vi "check limit channels.vi"(7 "RT Queues in":T8, 8 "Active channels":dbl[][](array[numeric]), 10 "Data":T1={"Parameters"={"FPGA Ref"=refnum, "data stream"={"data writer name"="error writer", "NS write buffer size"=16, "NS Buffer length"=0}, "FIFO Depth"=0, "Channel controls"={"FIFO channel count"=0, "active indices"=[], "active channels"=0, "channelScaling"=[], "scanivalveCount"=0, "channels"=[]}, "safetyChannels"={"oilP"=0, "airP"=0, "water"=0, "channelLimits"=[]}, "speedChannel"=0, "maxSpeedLimit"=0.0, "Torque"={"fixedOffset"=0.0, "filter"=FALSE, "fallingEdge"=FALSE, "swapEncoders"=FALSE}}, "Variables"={"Intermediary buffer"=[], "buffer position"=0, "write loop counter"=0, "NS write trigger"=0, "NS Connection status"=FALSE, "waiting for NS"=FALSE, "labAmbient"={"pressure"=0.0, "temperature"=0.0}, "scanivalvePorts"=[], "scanivalvePressures"=[], "data stream"="", "activeChannelLimitIndex"=[], "runningSpeedLimit"=0.0, "speedChannelIndex"=0, "Interlocks"={"gearboxOil"=FALSE, "bearingOil"=FALSE, "gearboxAir"=FALSE}, "interlockChannels"={"gearboxOil"=0, "bearingOil"=0, "air"=0}, "limitStates"=[]}}) -> (2 "Data out":T1={"Parameters"={"FPGA Ref"=refnum, "data stream"={"data writer name"="error writer", "NS write buffer size"=16, "NS Buffer length"=0}, "FIFO Depth"=0, "Channel controls"={"FIFO channel count"=0, "active indices"=[], "active channels"=0, "channelScaling"=[], "scanivalveCount"=0, "channels"=[]}, "safetyChannels"={"oilP"=0, "airP"=0, "water"=0, "channelLimits"=[]}, "speedChannel"=0, "maxSpeedLimit"=0.0, "Torque"={"fixedOffset"=0.0, "filter"=FALSE, "fallingEdge"=FALSE, "swapEncoders"=FALSE}}, "Variables"={"Intermediary buffer"=[], "buffer position"=0, "write loop counter"=0, "NS write trigger"=0, "NS Connection status"=FALSE, "waiting for NS"=FALSE, "labAmbient"={"pressure"=0.0, "temperature"=0.0}, "scanivalvePorts"=[], "scanivalvePressures"=[], "data stream"="", "activeChannelLimitIndex"=[], "runningSpeedLimit"=0.0, "speedChannelIndex"=0, "Interlocks"={"gearboxOil"=FALSE, "bearingOil"=FALSE, "gearboxAir"=FALSE}, "interlockChannels"={"gearboxOil"=0, "bearingOil"=0, "air"=0}, "limitStates"=[]}})   [LabVIEW 2018]
uses:
  Type Defs/Data processing loop data.ctl
  Type Defs/FPGA reference.ctl
  PC/type defs/channelControl.ctl
  Type Defs/channelScalingTypes.ctl
  Type Defs/scalingMethods.ctl
  ICL-LabVIEW_General/data channels/parent class/Data Channel.lvclass
  PC/type defs/channelLimitControl.ctl
  PC/type defs/limitActions.ctl
  Type Defs/Queues cluster.ctl
  ICL-LabVIEW_General/Message Scheduler/message scheduler.lvclass
  Queue VIs/En-queue RT message element.vi
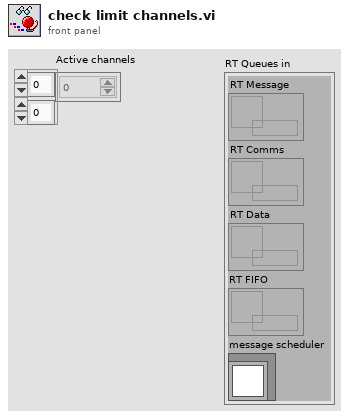
[diagram p1: front panel]
types:
  T1 = typedef "Data processing loop data.ctl" = cluster{"Parameters":cluster{"FPGA Ref":T2, "data stream":cluster{"data writer name":string, "NS write buffer size":i32, "NS Buffer length":u32}, "FIFO Depth":u32, "Channel controls":cluster{"FIFO channel count":i32, "active indices":i16[], "active channels":i32, "channelScaling":T3[], "scanivalveCount":i32, "channels":refnum<class "Data Channel.lvclass">[]}, "safetyChannels":cluster{"oilP":u16, "airP":u16, "water":u16, "channelLimits":T6[]}, "speedChannel":i32, "maxSpeedLimit":dbl, "Torque":cluster{"fixedOffset":dbl, "filter":bool, "fallingEdge":bool, "swapEncoders":bool}}, "Variables":cluster{"Intermediary buffer":dbl[][], "buffer position":u32, "write loop counter":u16, "NS write trigger":u32, "NS Connection status":bool, "waiting for NS":bool, "labAmbient":cluster{"pressure":dbl, "temperature":dbl}, "scanivalvePorts":u16[], "scanivalvePressures":dbl[], "data stream":refnum<k21>, "activeChannelLimitIndex":u16[], "runningSpeedLimit":dbl, "speedChannelIndex":i32, "Interlocks":cluster{"gearboxOil":bool, "bearingOil":bool, "gearboxAir":bool}, "interlockChannels":cluster{"gearboxOil":i32, "bearingOil":i32, "air":i32}, "limitStates":cluster{"warn":bool, "alarm":bool}[]}}
  T2 = typedef "FPGA reference.ctl" = refnum<k20>
  T3 = typedef "channelControl.ctl" = cluster{"index":u16, "active":bool, "channelType":T4, "module":u16, "terminal":u16, "channelName":string, "scalingMethod":T5, "scalingParameters":dbl[], "scaledUnits":string, "tempOffset":dbl}
  T4 = typedef "channelScalingTypes.ctl" = enum16{"calculation", "measurement", "scanivalve", "output", "digital"}
  T5 = typedef "scalingMethods.ctl" = enum16{"none", "linear", "thermocouple", "polynomial", "encoder", "RTD"}
  T6 = typedef "channelLimitControl.ctl" = cluster{"channelID":u16, "Enabled":bool, "warnValue":dbl, "limitValue":dbl, "Invert":bool, "limitAction":T7}
  T7 = typedef "limitActions.ctl" = enum16{"stop", "shutdown", "ignore"}
  T8 = typedef "Queues cluster.ctl" = cluster{"RT Message":refnum<queue>, "RT Comms":refnum<queue>, "RT Data":refnum<queue>, "RT FIFO":refnum<queue>, "message scheduler":refnum<class "message scheduler.lvclass">}
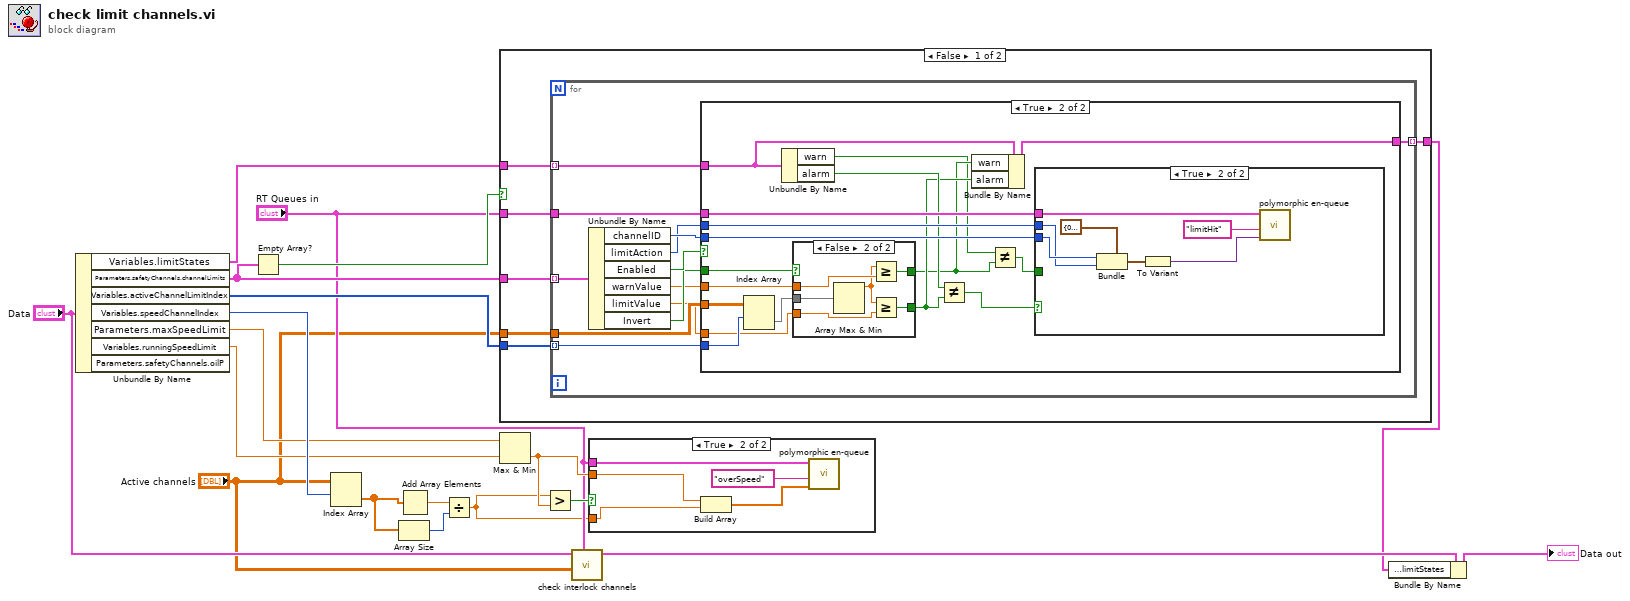
[diagram p0: block diagram]
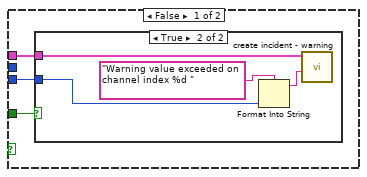
[diagram p4: hidden frame]
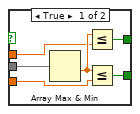
[diagram p6: hidden frame]
diagram:
  n1 = Unbundle By Name("Data") -> ("Variables.limitStates"=w3:cluster{"warn":bool, "alarm":bool}[], "Parameters.safetyChannels.channelLimits"=w18:T6[], "Variables.activeChannelLimitIndex"=w19:u16[], "Variables.speedChannelIndex"=w16:i32, "Parameters.maxSpeedLimit"=w15:dbl, "Variables.runningSpeedLimit"=w14:dbl)  [unwired: 1 out]
  n2 = Empty Array?(array=w18) -> (empty?=w17:bool)
  n3 = Index Array(array="Active channels", index (row)=w16) -> (element=w6:dbl[])  [unwired: 1 in]
  n4 = Array Size(array=w6) -> (size(s)=w5:i32)
  n5 = Add Array Elements(numeric array=w6) -> (sum=w7:dbl)
  n6 = Divide(x=w7, y=w5) -> (x/y=w4:dbl)
  n7 = case shown="False" w17 {
    tunnel: w19 -> [w25 _]
    tunnel: w18 -> [w24 _]
    tunnel: "Active channels" -> [w23 _]
    tunnel: "RT Queues in" -> [w22 _]
    tunnel: w3 -> [w21 w82]
    tunnel: [w20 w82] -> w1
    frame False {
      n8 = for {
        tunnel: w24 -> [w37] mode=indexing
        tunnel: w25 -> [w35] mode=indexing
        tunnel: w23 -> [w36]
        tunnel: w22 -> [w29]
        tunnel: w21 -> [w27] mode=indexing
        tunnel: [w26] -> w20 mode=indexing
        n9 = Unbundle By Name(w37) -> ("channelID"=w30:u16, "limitAction"=w28:T7, "Enabled"=w34:bool, "warnValue"=w31:dbl, "limitValue"=w32:dbl, "Invert"=w33:bool)
        n10 = case shown="True" w34 {
          tunnel: w36 -> [_ w55]
          tunnel: w35 -> [_ w54]
          tunnel: w33 -> [_ w53]
          tunnel: w32 -> [_ w51]
          tunnel: w31 -> [_ w50]
          tunnel: w30 -> [_ w48]
          tunnel: w28 -> [_ w47]
          tunnel: w29 -> [_ w49]
          tunnel: w27 -> [w38 w46]
          tunnel: [w38 w43] -> w26
          frame False {
          }
          frame True {
            n11 = Index Array(array=w55, index (row)=w54) -> (element=w52:dbl[])  [unwired: 1 in]
            n12 = Unbundle By Name(w46) -> ("warn"=w40:bool, "alarm"=w45:bool)
            n13 = case shown="False" w53 {
              tunnel: w52 -> [w74 w81]
              tunnel: w51 -> [w75 w78]
              tunnel: w50 -> [w72 w80]
              tunnel: [w71 w76] -> w42
              tunnel: [w70 w79] -> w41
              frame True {
                n14 = Array Max & Min(array=w74) -> (min value=w73:dbl)  [unwired: 3 out]
                n15 = Less Or Equal?(x=w73, y=w72) -> (x <= y?=w70:bool)
                n16 = Less Or Equal?(x=w73, y=w75) -> (x <= y?=w71:bool)
              }
              frame False {
                n17 = Array Max & Min(array=w81) -> (max value=w77:dbl)  [unwired: 3 out]
                n18 = Greater Or Equal?(x=w77, y=w80) -> (x >= y?=w79:bool)
                n19 = Greater Or Equal?(x=w77, y=w78) -> (x >= y?=w76:bool)
              }
            }
            n20 = Not Equal?(x=w45, y=w42) -> (x != y?=w44:bool)
            n21 = Bundle By Name(cluster=w46, "warn"=w41, "alarm"=w42) -> (w43:cluster{"warn":bool, "alarm":bool})
            n22 = Not Equal?(x=w40, y=w41) -> (x != y?=w39:bool)
            n23 = case shown="True" w44 {
              tunnel: w39 -> [w58 _]
              tunnel: w49 -> [w57 w63]
              tunnel: w48 -> [w56 w65]
              tunnel: w47 -> [_ w64]
              frame False {
                n24 = case shown="True" w58 {
                  tunnel: w57 -> [_ w60]
                  tunnel: w56 -> [_ w59]
                  frame False {
                  }
                  frame True {
                    n25 = Format Into String(format string="Warning value exceeded on channel index %d ", w59) -> (resulting string=w61:string)  [unwired: 2 in, 1 out]
                    n26 = call "create incident - warning.vi"("warning description"=w61, "RT Queues"=w60) -> ()  [unwired: 9 in, 1 out]
                  }
                }
              }
              frame True {
                n27 = Bundle(cluster=cluster{"channelID":u16, "limitAction":T7} {"channelID"=0, "limitAction"=enum."stop"}, "channelID"=w65, "limitAction"=w64) -> (w67:cluster{"channelID":u16, "limitAction":T7})
                n28 = To Variant(anything=w67) -> (Variant=w69:variant)
                n29 = call-poly "polymorphic en-queue.vi"("Data"=w69, "Message"="limitHit", "RT Queues"=w63) -> ()  [unwired: 8 in, 1 out]
              }
            }
          }
        }
      }
    }
    frame True {
    }
  }
  n30 = Max & Min(x=w15, y=w14) -> (min(x,y)=w13:dbl)  [unwired: 1 out]
  n31 = Greater?(x=w4, y=w13) -> (0:w12:bool)
  n32 = call "check interlock channels.vi"("RT Queues in"="RT Queues in", "scaledData"="Active channels", "Data in"="Data") -> ("Data out"=w11:T1)  [unwired: 8 in]
  n33 = case shown="True" w12 {
    tunnel: "RT Queues in" -> [_ w85]
    tunnel: w13 -> [_ w86]
    tunnel: w4 -> [_ w83]
    frame False {
    }
    frame True {
      n34 = Build Array(w86, w83) -> (w84:dbl[])
      n35 = call-poly "polymorphic en-queue.vi"("Data"=w84, "Message"="overSpeed", "RT Queues"=w85) -> ()  [unwired: 8 in, 1 out]
    }
  }
  n36 = Bundle By Name(cluster=w11, "Variables.limitStates"=w1) -> (→"Data out":T1)
